vi "Read Encoder.vi"(11 "ValveModbus in":refnum<class "ValveModbus.lvclass">) -> (2 "Encoder":i32, 3 "ValveModbus out":refnum<class "ValveModbus.lvclass">)   [LabVIEW 2019, in "ValveModbus.lvclass"]
uses:
  ValveModbus.lvclass
  ValveModbus.lvclass/ValveModbus.ctl
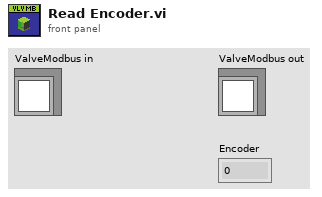
[diagram p1: front panel]
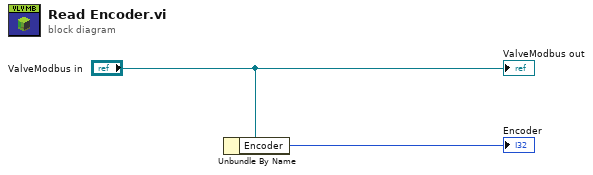
[diagram p0: block diagram]
diagram:
  n1 = Unbundle By Name("ValveModbus in") -> ("Encoder"=→"Encoder":i32)
  "ValveModbus out" <- "ValveModbus in"
